vi "HIL Simulation and Testing.vi"() -> ()   [LabVIEW 2021]
uses:
  <vilib>/Simulation/Scripting/Companion Diagram/SimConfigNode/SimParams.ctl
  <vilib>/Simulation/Scripting/Companion Diagram/SimConfigNode/_simSolvers.ctl
  <vilib>/Simulation/Implementation/Shared/SIMSCR Execution Mode.ctl
  <vilib>/Simulation/Param Hierarchy/Typedefs/SIMPH Param Control Actions.ctl
  <vilib>/Simulation/Implementation/Shared/NILVSim_ParamChanged.vi
  <vilib>/Simulation/Implementation/Shared/NILVSIM_BeginStep.vi
  <vilib>/Simulation/Implementation/Shared/NILVSim_Manager.vi
  <vilib>/Utility/error.llb/Clear Errors.vi
  <vilib>/Simulation/Implementation/Shared/NILVSim_FinalizeModel.vi
  <vilib>/Simulation/Implementation/Shared/SIM Unbundle Sim Info.vi
  <vilib>/Simulation/Implementation/Shared/NILVSim_Initialize.vi
  <vilib>/Simulation/Utility/Implementation/NILVSim Get Time and IsAcceptedStep.vi
  <vilib>/Simulation/Implementation/Shared/SIMSH Read Queue.vi
  <vilib>/Simulation/Implementation/Shared/NILVSim_GetModelError.vi
  <vilib>/Simulation/Implementation/Shared/SIM Bundle Sim Info.vi
  <vilib>/Simulation/Implementation/XNodeFramework/SimXNode/SimX.xnode
  Blackbox/Air Heater Black Box Model.vi
  <vilib>/Simulation/Scripting/Companion Diagram/SimConfigNode/SimDog.xnode
  <vilib>/Simulation/Implementation/Shared/NI_SIM_Implementation.lvlib
panel:
  out "Control Value [V]":dbl format="%.2g"
  out "Temperature [°C]":dbl format="%.1g"
  out "Control Chart":dbl(graph)=1.1724378087907898
  out "Measurement Chart":dbl(graph)
  in  "Stop":bool
  # "Note! The Setpoint/Set Value (SV) is set on the Fuji PXG5 Hardware"
  # "Process Value (PV)"
  # "Manipulated Value (MV)"
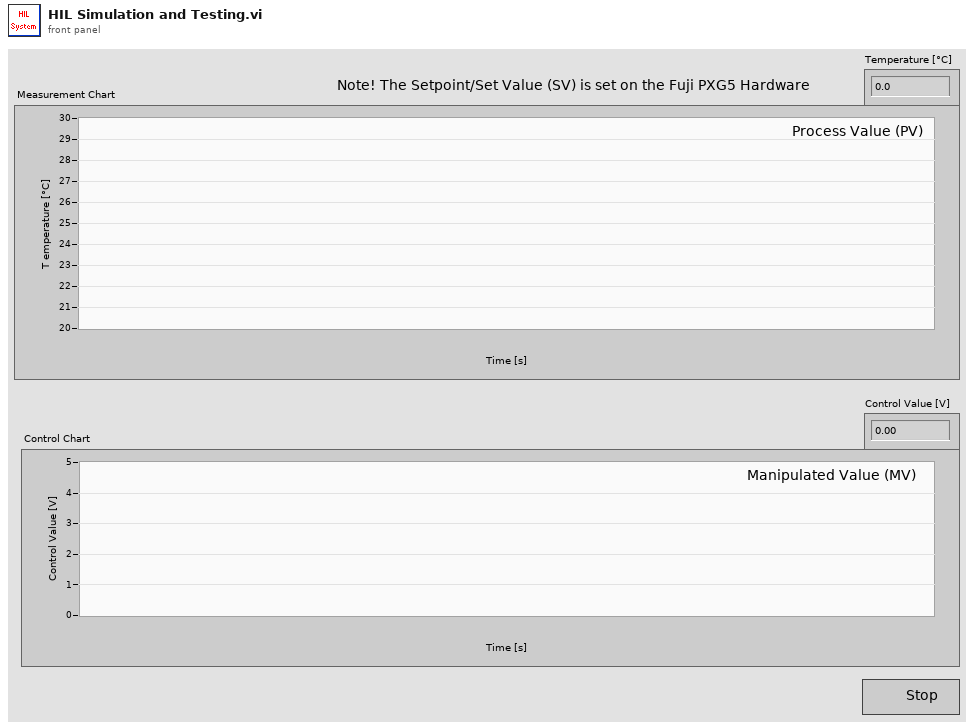
[diagram p1: front panel]
types:
  T1 = enum16{"Simulate to Completion", "Single Time-Step Simulation (Fixed Step Only)"}
  T2 = typedef "SIMSCR Execution Mode.ctl" = enum16{"Simulate to Completion", "Single Time-Step Simulation (Fixed Step Only)"}
  T3 = typedef "SIMPH Param Control Actions.ctl" = enum16{"get params", "set params"}
  T4 = cluster{"SIMSH Sim Time":dbl, "Linear Scaling with Points.vi 2":cluster{"Output":dbl}, "Select":cluster{"s? t:f":dbl}, "Summation 3":cluster{"Result":dbl}, "Square Root":cluster{"sqrt(x)":dbl}, "Gaussian White Noise PtByPt.vi":cluster{"Gaussian white noise":dbl}, "Integrator":cluster{"output":dbl}, "Multiplication":cluster{"Result":dbl}, "Summation":cluster{"Result":dbl}, "Multiplication 2":cluster{"Result":dbl}, "Transport Delay":cluster{"output":dbl}, "Summation 2":cluster{"Result":dbl}}
  T5 = typedef "SimParams.ctl" = cluster{"Initial Time (s)":dbl, "Final Time (s)":dbl, "Step Size (s)":dbl, "ODE Solver":T6, "Minimum Step Size (s)":dbl, "Maximum Step Size (s)":dbl, "Relative Tolerance":dbl, "Absolute Tolerance":dbl, "Software Timing":bool, "Initial Step Size (s)":dbl, "Automatic Fixed Step Size?":bool, "Automatic Discrete Step Size?":bool, "Discrete Step Size (s)":dbl, "Calculate using Time Step":bool, "Solver Wired?":bool, "Prev.Frm.Expected End":u64, "Prev.Frm.Actual End":u64, "Prev.Frm.Finished Late?":bool, "Prev.Iter.Expected End":u64, "Prev.Iter.Actual End":u64, "Prev.Iter.Finished Late?":bool, "Expected Iteration Start":u64, "Actual Iteration Start":u64, "Expected Frame Start":u64, "Actual Frame Start":u64, "Source Name":string, "Name":string, "Period":i64, "Deadline":i64, "Offset":i64, "Start":i64, "Priority":i32, "Timeout":i32, "Processor":i32, "Mode":enum32{"No Change", "Process missed periods, maintain original phase", "Discard missed periods, maintain original phase", "Process missed periods, ignore original phase", "Discard missed periods, ignore original phase"}, "Wakeup reason":enum32{"Normal", "Aborted", "Asynchronous wakeup", "Timing source error", "Timed loop error", "Timeout"}, "Error":errorcluster, "Source Type":string, "Secondary Source Type":string, "Global End Time":u64, "Global Start Time":u64, "Full Solver Reset":bool, "Execution Mode":T2, "Nan/Inf Check":bool, "Custom Solver Library":string, "Solver Is Variable":bool, "custom solver name":string, "Signal Collection Decimation":u32}
  T6 = typedef "_simSolvers.ctl" = enum16{"Runge-Kutta 1 (Euler)", "Runge-Kutta 2", "Runge-Kutta 3", "Runge-Kutta 4", "Runge-Kutta 23 (variable)", "Runge-Kutta 45 (variable)", "BDF (variable)", "Adams-Moulton (variable)", "Rosenbrock (variable)", "Discrete States Only", "SDIRK 4 (variable)", "Radau 5 (variable)", "Radau 9 (variable)", "Radau 13 (variable)", "Radau [Variable Order] (variable)", "Gear's Method (variable)", "Linearizer", "State Query", "Trim Eval", "Custom Solver"}
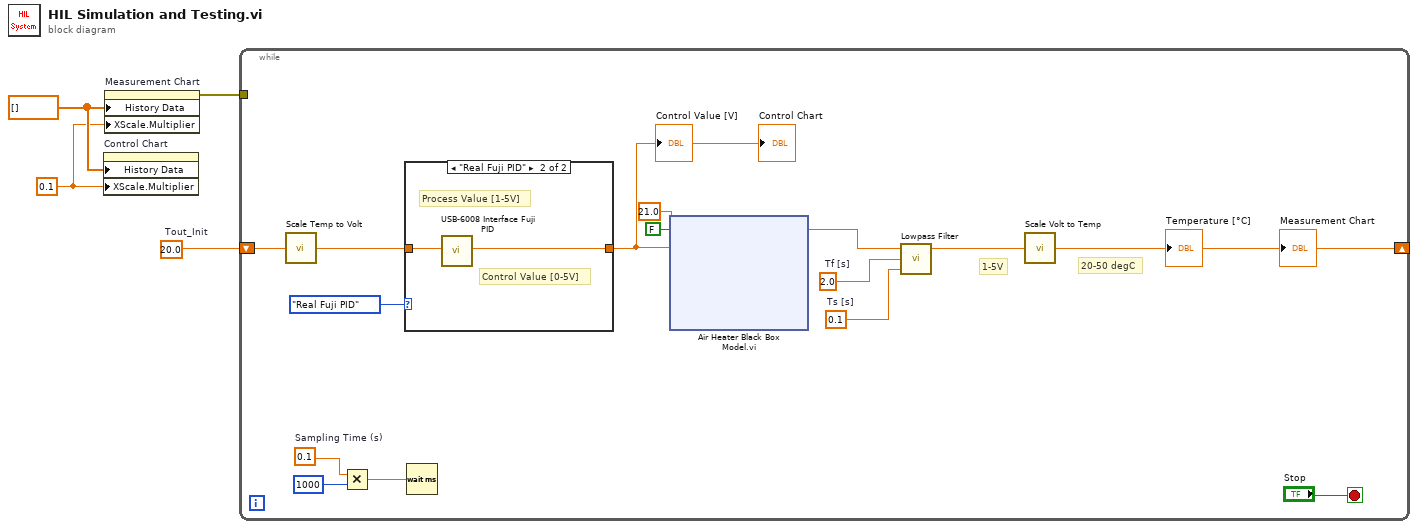
[diagram p0: block diagram]
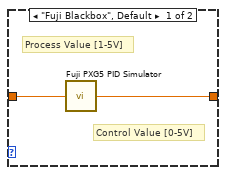
[diagram p2: hidden frame]
diagram:
  w4 = 20.0  # Tout_Init
  w2 = 0.1 ("X Scale.Offset and Multiplier:Multiplier")
  w3 = dbl[] [] ("History Data")
  n1 = property on="Control Chart" class="WFChart (strict)"("History Data"=w3, "XScale.Multiplier"=w2) -> ()  [unwired: 2 in, 2 out]
  n2 = property on="Measurement Chart" class="WFChart (strict)"("History Data"=w3, "XScale.Multiplier"=w2) -> (error out=w1:errorcluster)  [unwired: 2 in, 1 out]
  n3 = while {
    shift-right: [w10] -> _
    shift-left: w4 -> [w8]
    tunnel: w1 -> [_]
    stop <- "Stop" stop-if-true
    w14 = 0.1  # Ts [s]
    w15 = 2.0  # Tf [s]
    w16 = 0.1  # Sampling Time (s)
    # "1-5V"
    # "20-50 degC"
    n4 = call "Scale Temp to Volt.vi"("Input Value [20-50degC]"=w8) -> ("Output Value [1-5V]"=w7:dbl)
    n5 = Multiply(x=w16, y=1000) -> (x*y=w18:dbl)
    n6 = case shown="\"Real Fuji PID\"" enum16{"Fuji Blackbox", "Real Fuji PID"}."Real Fuji PID" ("Enum") {
      tunnel: [w21 w22] -> w12
      tunnel: w7 -> [w20 w23]
      frame "Fuji Blackbox", Default {
        # "Process Value [1-5V]"
        # "Control Value [0-5V]"
        n7 = call "Fuji PXG5 PID Simulator.vi"("Input (1-5V)"=w20) -> ("Output (0-5V)"=w21:dbl)
      }
      frame "Real Fuji PID" {
        # "Process Value [1-5V]"
        # "Control Value [0-5V]"
        n8 = call "USB-6008 Interface Fuji PID.vi"("Process Value  [1-5V]"=w23) -> ("Control Value [0-5V]"=w22:dbl)
      }
    }
    "Control Chart" <- w12
    "Control Value [V]" <- w12
    n9 = Wait (ms)(milliseconds to wait=w18) -> ()  [unwired: 1 out]
    n10 = xnode "Air Heater Black Box Model.vi"("Noise"=FALSE, "T_env [C]"=21.0, "Control Signal [0-5V]"=w12) -> ("Tout [1-5V]"=w13:dbl)  [unwired: 2 in, 1 out]
    n11 = call "Lowpass Filter.vi"("Ts [s]"=w14, "Tf [s]"=w15, "Filter Input"=w13) -> ("Filter Output"=w11:dbl)
    n12 = call "Scale Volt to Temp.vi"("Input Value [1-5V]"=w11) -> ("Output Value [20-50degC]"=w10:dbl)
    "Measurement Chart" <- w10
    "Temperature [°C]" <- w10
  }
